vi "NewNYStyleCheesePizza.vi"(8 "error in (no error)":errorcluster) -> (0 "error out":errorcluster, 3 "NYStyleCheesePizza":refnum<class "NYStyleCheesePizza.lvclass">)   [LabVIEW 2020, in "FactoryMethod.lvlib" / "PizzaFactoryMethod.lvlib" / "NYStyleCheesePizza.lvclass"]
uses:
  NYStyleCheesePizza.lvclass
  NYStyleCheesePizza.lvclass/NYStyleCheesePizza.ctl
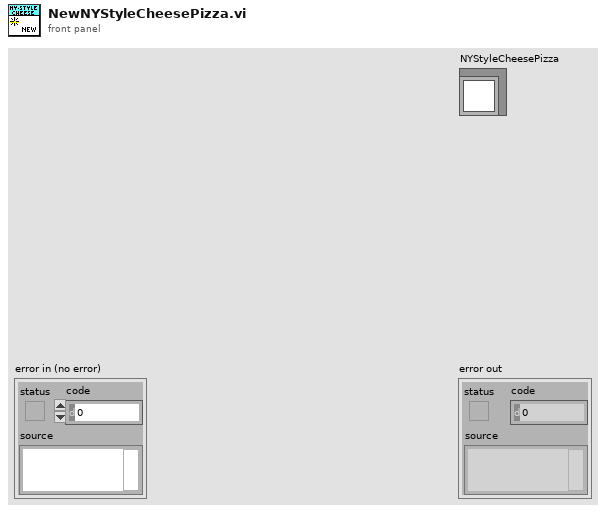
[diagram p1: front panel]
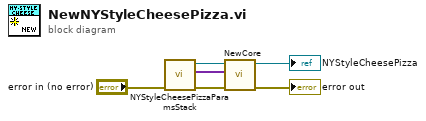
[diagram p0: block diagram]
diagram:
  n1 = call "NYStyleCheesePizzaParamsStack.vi"("error iN"="error in (no error)") -> ("error out"=w6:errorcluster, "HierarchyParams"=w5:variant[], "NYStyleCheesePizza"=w1:refnum<class "NYStyleCheesePizza.lvclass">)  [unwired: 8 in]
  n2 = call-dynamic "NewCore.vi"("error in (no error)"=w6, "ParamsArray"=w5, "NYStyleCheesePizza"=w1) -> ("error out"=→"error out":errorcluster, "NYStyleCheesePizza"=→"NYStyleCheesePizza":refnum<class "NYStyleCheesePizza.lvclass">)  [unwired: 7 in]
